vi "GetType.vi"(8 "error in (no error)":errorcluster, 11 "Clear Records Msg":refnum<class "Clear Records Msg.lvclass">) -> (0 "error out":errorcluster, 2 "Data Sample":variant, 3 "Clear Records Msg":refnum<class "Clear Records Msg.lvclass">)   [LabVIEW 2015, in "CS++MCS.lvlib" / "Clear Records Msg.lvclass"]
uses:
  Clear Records Msg.lvclass
  Clear Records Msg.lvclass/Clear Records Msg.ctl
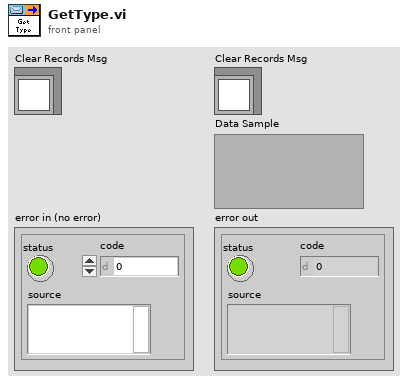
[diagram p1: front panel]
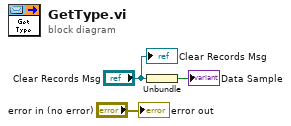
[diagram p0: block diagram]
diagram:
  n1 = Unbundle("Clear Records Msg") -> (→"Data Sample":bool)
  "error out" <- "error in (no error)"
  "Clear Records Msg" <- "Clear Records Msg"
